vi "Resolve M.vi"(11 "待解析数据":string) -> (3 "M区数据":bool[](array[boolean]))   [LabVIEW 2014]
panel:
  out "字符串 2":string
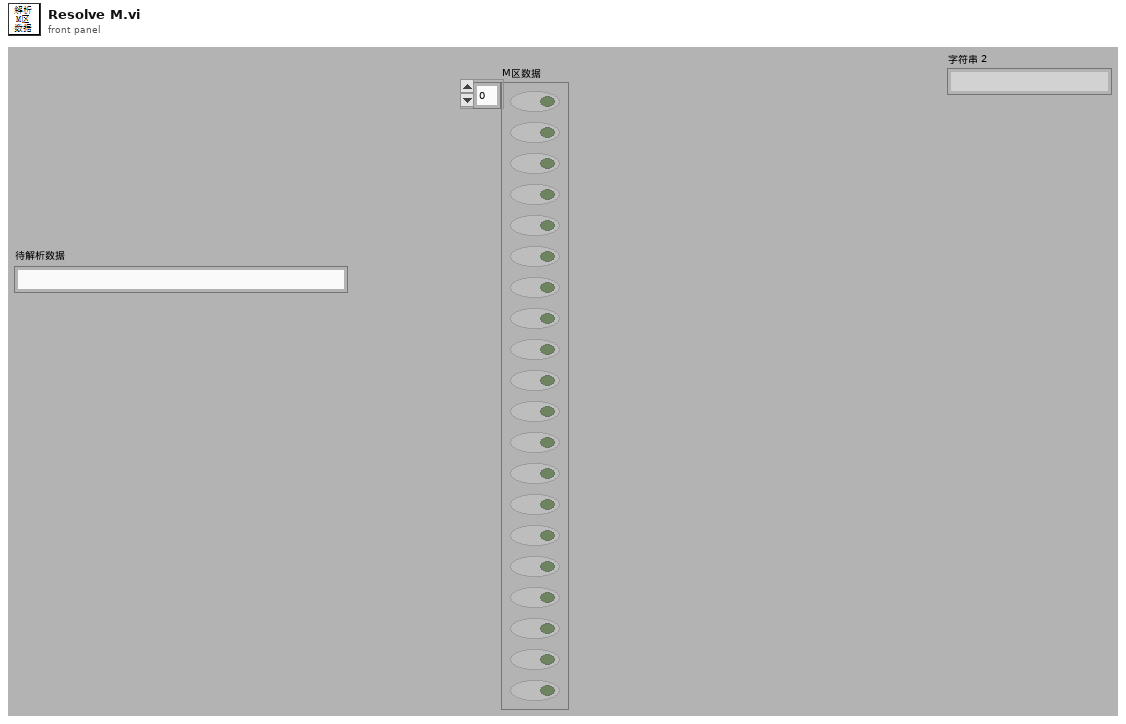
[diagram p1: front panel]
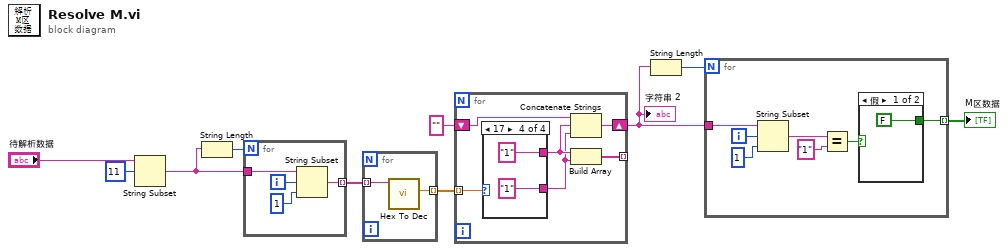
[diagram p0: block diagram]
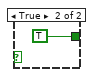
[diagram p2: hidden frame]
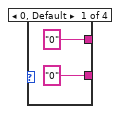
[diagram p3: hidden frame]
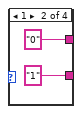
[diagram p4: hidden frame]
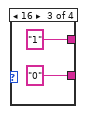
[diagram p5: hidden frame]
diagram:
  n1 = String Subset(string="待解析数据", offset (0)=11 ("偏移量(0)")) -> (substring=w3:string)  [unwired: 1 in]
  n2 = String Length(string=w3) -> (length=w9:i32)
  n3 = for {
    N: w9 -> [_]
    tunnel: [w12] -> w8 mode=indexing
    tunnel: w3 -> [w11]
    i -> [w14]
    n4 = String Subset(string=w11, offset (0)=w14, length (rest)=1 ("长度（剩余）")) -> (substring=w12:string)
  }
  n5 = for {
    tunnel: w8 -> [w16] mode=indexing
    tunnel: [w15] -> w10 mode=indexing
    n6 = call "Hex To Dec.vi"("十六进制字符串"=w16) -> ("十进制整数"=w15:dbl)  [unwired: 7 in, 3 out]
  }
  n7 = for {
    tunnel: w10 -> [w22] mode=indexing
    tunnel: [w19] -> _ mode=indexing
    shift-right: [w17] -> w6
    shift-left: "" -> [w18]
    n8 = case shown="17" w22 {
      tunnel: ["0" "0" "1" "1"] -> w21
      tunnel: ["0" "1" "0" "1"] -> w20
      frame 0, Default {
      }
      frame 1 {
      }
      frame 16 {
      }
      frame 17 {
      }
    }
    n9 = Concatenate Strings(w18, w21, w20) -> (w17:string)
    n10 = Build Array(w21, w20) -> (w19:string[])
  }
  "字符串 2" <- w6
  n11 = String Length(string=w6) -> (length=w7:i32)
  n12 = for {
    N: w7 -> [_]
    tunnel: w6 -> [w34]
    tunnel: [w35] -> w5 mode=indexing
    i -> [w33]
    n13 = String Subset(string=w34, offset (0)=w33, length (rest)=1 ("长度（剩余）")) -> (substring=w31:string)
    n14 = Equal?(x=w31, y="1") -> (x = y?=w37:bool)
    n15 = case shown="假" w37 {
      tunnel: [FALSE TRUE] -> w35
      frame False {
      }
      frame True {
      }
    }
  }
  "M区数据" <- w5
